vi "Becker-Hickl Load .sdt FLI Dataset Information.vi"(8 "error in (no error)":errorcluster, 11 "File Path":path) -> (0 "error out":errorcluster, 1 "Data Description":string, 2 "Metadata":string, 3 "FLI Data File Information":T1, 4 "Load Time (s)":dbl)   [LabVIEW 2021, in "Becker-Hickl Files.lvlib"]
uses:
  Becker-Hickl Files.lvlib
  AlliGator/AlliGator FLI Data File Information.ctl
  Phasor/Phasor Fluorescence Lifetime Parameters v3.ctl
  AlliGator/AlliGator FLI Dataset Type.ctl
  Load Single Gate Image from Becker-Hickl .sdt File.vi
  AlliGator/AlliGator Files.lvlib
  AlliGator/AlliGator HDF5.lvlib
  Phasor/Phasor.lvlib
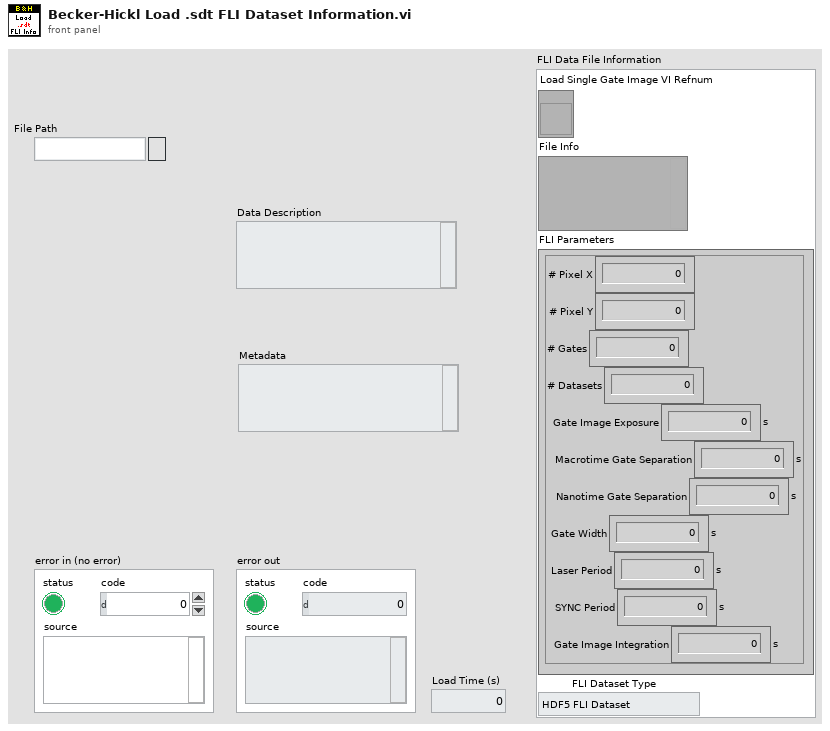
[diagram p1: front panel]
types:
  T1 = typedef "AlliGator HDF5.lvlib/AlliGator FLI Data File Information.ctl" = cluster{"Load Single Gate Image VI Refnum":refnum<vi>, "File Info":variant, "FLI Parameters":T2, "FLI Dataset Type":T3}
  T2 = typedef "Phasor.lvlib/Phasor Fluorescence Lifetime Parameters v3.ctl" = cluster{"# Pixel X":i32, "# Pixel Y":i32, "# Gates":i32, "# Datasets":i32, "Gate Image Exposure":dbl[unit], "Macrotime Gate Separation":dbl[unit], "Nanotime Gate Separation":dbl[unit], "Gate Width":dbl[unit], "Laser Period":dbl[unit], "SYNC Period":dbl[unit], "Gate Image Integration":dbl[unit]}
  T3 = typedef "AlliGator Files.lvlib/AlliGator FLI Dataset Type.ctl" = enum16{"HDF5 FLI Dataset", "Gate Image Folder", ".sdt FLI Dataset (Becker & Hickl)", ".ptu FLI Dataset (PicoQuant)", "SS1 FLI Dataset", "SS2 FLI Dataset", "I/m/phi Dataset", ".bin FLI Dataset (PicoQuant Binned)", ".bin FLI Dataset (Piccolo Binned)"}
  T4 = typedef "Becker-Hickl Files.lvlib/Becker-Hickl File Information.ctl" = cluster{"Information String":string, "File Header":T5, "Image Parameters":T6, "TAC Parameters":T7, "Measurement Information":T8, "File Path":path}
  T5 = typedef "Becker-Hickl Files.lvlib/Becker-Hickl File Header Structure.ctl" = cluster{"Revision":i16, "Info Offset":i32, "Info Length":i16, "Setup Offset":i32, "Setup Length":i16, "Data Block Offset":i32, "# Data Blocks":i16, "Data Block Length":i32, "Measurement Description Block Offset":i32, "# Measurement Description Blocks":i16, "Measurement Description Length":i16, "Header Valid":u16, "Reserved 1":u32, "Reserved 2":u16, "Checksum":u16}
  T6 = typedef "Becker-Hickl Files.lvlib/Becker-Hickl Image Parameters.ctl" = cluster{"Pixel T (s)":dbl, "Scan X":i32, "Scan Y":i32, "Image X":i32, "Image Y":i32}
  T7 = typedef "Becker-Hickl Files.lvlib/Becker-Hickl TAC Parameters.ctl" = cluster{"Frequency (Hz)":dbl, "Frequency Divider":i32, "TAC Range (s)":dbl, "TAC Gain":i32, "TAC Offset (%)":dbl, "TAC Limit Low (%)":dbl, "TAC Limit High (%)":dbl, "TAC Bin (s)":dbl, "ADC bins":i32, "Histogram Range (s)":dbl}
  T8 = typedef "Becker-Hickl Files.lvlib/Becker-Hickl Measurement Information.ctl" = cluster{"Measurement Stop Info":T9, "Measurement FCS Info":T10, "Addl Histogram Measurement Info":T11, "Creation Time":string, "Creation Date":string, "Module Serial Number":string, "Measurement Mode":i16, "CFD LL":sgl, "CFD LH":sgl, "CFD ZC":sgl, "CFD HF":sgl, "SYN ZC":sgl, "SYN FD":i16, "SYN HF":sgl, "TAC R":sgl, "TAC G":i16, "TAC OF":sgl, "TAC LL":sgl, "TAC LH":sgl, "ADC RE":i16, "EAL DE":i16, "NCX":i16, "NCY":i16, "Page":u16, "Col T":sgl, "Rep T":sgl, "Stop T":i16, "Overflow":u8, "Use Motor":i16, "Steps":u16, "Offset":sgl, "Dither":i16, "Increment":i16, "Memory Bank":i16, "Module Type":string, "SYN Th":sgl, "Dead Time Compensation":i16, "Polarity L":i16, "Polarity F":i16, "Polarity P":i16, "Line Divider":i16, "Accumulate":i16, "Flyback Y":i32, "Flyback X":i32, "Border U":i32, "Border L":i32, "Pixel Time":sgl, "Pixel Clock":i16, "Trigger":i16, "Scan X":i32, "Scan Y":i32, "Scan RX":i32, "Scan RY":i32, "FIFO Type":i16, "Exp Divider":i32, "Module Type Code":u16, "Module FPGA Version":u16, "Overflow Corr Factor":sgl, "ADC Zoom":i32, "Cycles":i32, "Image X":i32, "Image Y":i32, "Image RX":i32, "Image RY":i32, "XY Gain":i16, "Master Clock":i16, "ADC Delay":i16, "Detector Type":i16, "X Axis":i16}
  T9 = typedef "Becker-Hickl Files.lvlib/Becker-Hickl Measurement Stop Info.ctl" = cluster{"Status":u16, "Flags":u16, "Stop Time":sgl, "Current Step":i32, "Current Cycle":i32, "Current Page":i32, "Min Sync Rate":sgl, "Min CFD Rate":sgl, "Min TAC Rate":sgl, "Min ADC Rate":sgl, "Max Sync Rate":sgl, "Max CFD Rate":sgl, "Max TAC Rate":sgl, "Max ADC Rate":sgl, "Reserved 1":i32, "Reserved 2":sgl}
  T10 = typedef "Becker-Hickl Files.lvlib/Becker-Hickl FCS Measurement Info.ctl" = cluster{"Channel":u16, "FCS Decay Calc":u16, "Macrotime Resolution (0.1 ns)":u32, "Correlation Time (ms)":sgl, "# Photons":u32, "# FCS Points":i32, "End Time":sgl, "# FIFO Overflows":u16, "FCS Type":u16, "# Cross FCS Channel":u16, "Module Number":u16, "Cross FCS Module Number":u16, "Cross FCS Macrotime Resolution (0.1 ns)":u32}
  T11 = typedef "Becker-Hickl Files.lvlib/Becker-Hickl Additional Histogram Measurement Info.ctl" = cluster{"FIDA Time (ms)":sgl, "FILDA Time (ms)":sgl, "# FIDA Points":i32, "# FILDA Points":i32, "MCS Time (ms)":sgl, "# MCS Points":i32, "# Cross FCS Photons":u32, "Reserved1":i32, "Reserved2":dbl, "Reserved3":dbl}
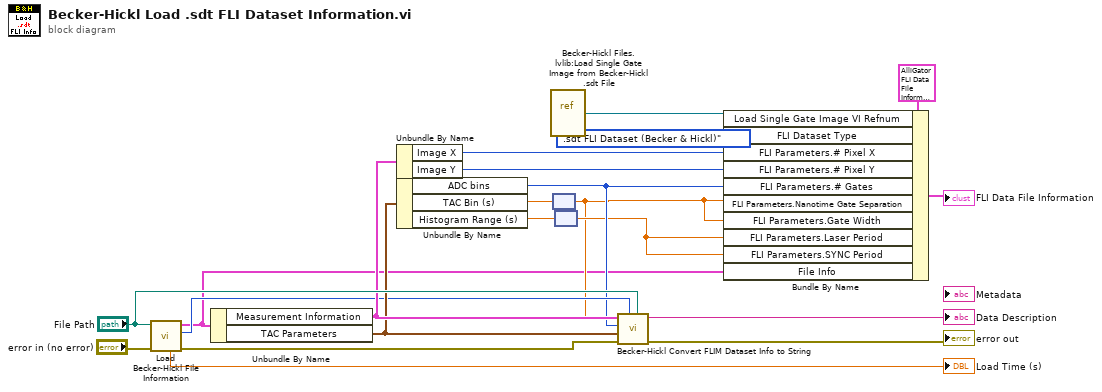
[diagram p0: block diagram]
diagram:
  n1 = call "Load Becker-Hickl File Information.vi"("Error In"="error in (no error)", "File Path Control"="File Path") -> ("Error Out"=w7:errorcluster, "Size (in Bytes)"=w8:i64, "B&H File Information"=w1:T4, "Load Time (s)"=→"Load Time (s)":dbl)  [unwired: 6 in]
  n2 = Unbundle By Name(w1) -> ("Measurement Information"=w11:T8, "TAC Parameters"=w10:T7)
  n3 = Unbundle By Name(w11) -> ("Image X"=w15:i32, "Image Y"=w14:i32)
  n4 = Unbundle By Name(w10) -> ("ADC bins"=w5:i32, "TAC Bin (s)"=w20:dbl, "Histogram Range (s)"=w21:dbl)
  n5 = vi-ref "Becker-Hickl Files.lvlib:Load Single Gate Image from Becker-Hickl .sdt File.vi"() -> (w2:refnum<vi>)
  n6 = node(w20) -> (w3:dbl[unit])
  n7 = node(w21) -> (w4:dbl[unit])
  n8 = call "Becker-Hickl Convert FLIM Dataset Info to String.vi"("File Path"="File Path", "Step Duration"=w3, "File Size"=w8, "error in (no error)"=w7, "TAC Parameters"=w10, "# Gates"=w5, "Measurement Information"=w11) -> ("Error Out"=→"error out":errorcluster, "Data Description"=→"Data Description":string)  [unwired: 3 in]
  n9 = Bundle By Name(cluster=T1 {"Load Single Gate Image VI Refnum"=refnum, "File Info"=variant, "FLI Parameters"={"# Pixel X"=0, "# Pixel Y"=0, "# Gates"=0, "# Datasets"=0, "Gate Image Exposure"=0.0, "Macrotime Gate Separation"=0.0, "Nanotime Gate Separation"=0.0, "Gate Width"=0.0, "Laser Period"=0.0, "SYNC Period"=0.0, "Gate Image Integration"=0.0}, "FLI Dataset Type"=enum."HDF5 FLI Dataset"} ("FLI Data File Information"), "Load Single Gate Image VI Refnum"=w2, "FLI Dataset Type"=AlliGator_FLI_Dataset_Type.".sdt FLI Dataset (Becker & Hickl)", "FLI Parameters.# Pixel X"=w15, "FLI Parameters.# Pixel Y"=w14, "FLI Parameters.# Gates"=w5, "FLI Parameters.Nanotime Gate Separation"=w3, "FLI Parameters.Gate Width"=w3, "FLI Parameters.Laser Period"=w4, "FLI Parameters.SYNC Period"=w4, "File Info"=w1) -> (→"FLI Data File Information":T1)
